vi "LoadGraphImage.vi"(11 "relative path":string) -> (0 "Y Scale.Range":T1={"Minimum"=0.0, "Maximum"=0.9, "Increment"=0.1, "Minor Increment"=0.01, "Start"=0.0}, 1 "X Scale.Range":T1={"Minimum"=0.0, "Maximum"=0.8, "Increment"=0.1, "Minor Increment"=0.01, "Start"=0.0}, 2 "PlotAreaSize":T2, 3 "picture":picture)   [LabVIEW 2011]
uses:
  <vilib>/Utility/miscctls.llb/LVBoundsTypeDef.ctl
  <vilib>/Utility/miscctls.llb/LVRangeTypeDef.ctl
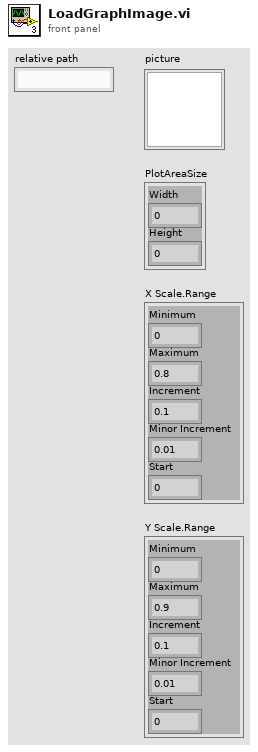
[diagram p1: front panel]
types:
  T1 = typedef "LVRangeTypeDef.ctl" = cluster{"Minimum":dbl, "Maximum":dbl, "Increment":dbl, "Minor Increment":dbl, "Start":dbl}
  T2 = typedef "LVBoundsTypeDef.ctl" = cluster{"Width":u32, "Height":u32}
  T3 = typedef "imagedata.ctl" = cluster{"image type":i32, "image depth":i32, "image":u8[], "mask":u8[], "colors":u32[], "Rectangle":cluster{"left":i16, "top":i16, "right":i16, "bottom":i16}}
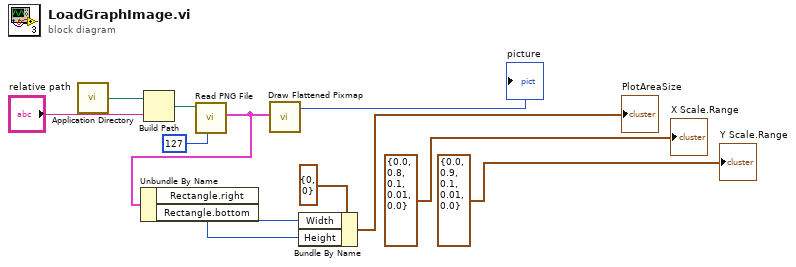
[diagram p0: block diagram]
diagram:
  n1 = call <vilib>:"Application Directory.vi"() -> ("Application Directory"=w3:path)
  n2 = Build Path(base path=w3, name or relative path="relative path") -> (appended path=w2:path)
  n3 = call <vilib>:"Read PNG File.vi"("Transparency Thresh"=u8 127, "path to PNG file"=w2) -> ("image data"=w9:T3)  [unwired: 7 in, 2 out]
  n4 = Unbundle By Name(w9) -> ("Rectangle.right"=w6:i16, "Rectangle.bottom"=w5:i16)
  n5 = call <vilib>:"Draw Flattened Pixmap.vi"("image data"=w9) -> ("new picture"=→"picture":picture)  [unwired: 8 in]
  n6 = Bundle By Name(cluster=T2 {"Width"=0, "Height"=0} ("Plot Area:Size"), "Width"=w6, "Height"=w5) -> (→"PlotAreaSize":T2)
  "X Scale.Range" <- T1 {"Minimum"=0.0, "Maximum"=0.8, "Increment"=0.1, "Minor Increment"=0.01, "Start"=0.0} ("X Scale.Range")
  "Y Scale.Range" <- T1 {"Minimum"=0.0, "Maximum"=0.9, "Increment"=0.1, "Minor Increment"=0.01, "Start"=0.0} ("Y Scale.Range")
